vi "题目6.vi"() -> ()   [LabVIEW 2017]
panel:
  out "字符串":string
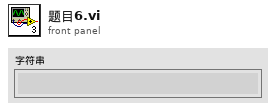
[diagram p1: front panel]
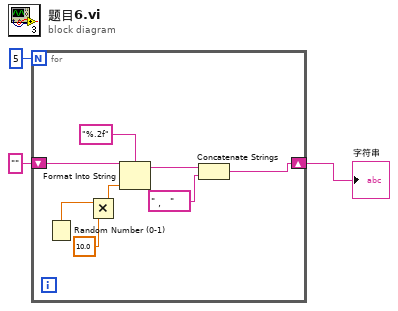
[diagram p0: block diagram]
diagram:
  n1 = for {
    N: 5 -> [_]
    shift-right: [w5] -> w2
    shift-left: "" -> [w4]
    n2 = Random Number (0-1)() -> (number: 0 to 1=w8:dbl)
    n3 = Multiply(x=w8, y=10.0) -> (x*y=w9:dbl)
    n4 = Format Into String(format string="%.2f" ("格式字符串"), initial string=w4, w9) -> (resulting string=w11:string)  [unwired: 1 in, 1 out]
    n5 = Concatenate Strings(w11, "，  " ("字符串")) -> (w5:string)
  }
  "字符串" <- w2
